vi "质控报警信息.vi"(11 "data in":T1) -> ()   [LabVIEW 2016, in "质控单元.lvlib"]
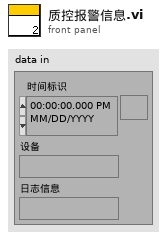
[diagram p1: front panel]
types:
  T1 = cluster{"时间标识":timestamp, "设备":string, "日志信息":string}
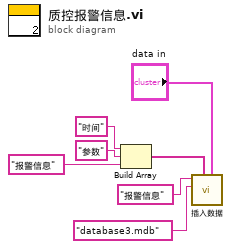
[diagram p0: block diagram]
diagram:
  n1 = Build Array("时间", "参数" ("元素"), "报警信息") -> (w4:string[])
  n2 = call "插入数据.vi"("data"="data in", "columns"=w4, "database"="database3.mdb", "table"="报警信息") -> ()  [unwired: 7 in, 1 out]
